vi "Clean up VI.vi"() -> ()   [LabVIEW 2013]
doc: "This .vi recenters the front panel \"pane\" to the origin, and adjusts the size of the window to fit the controls.\nIt also does the same with the block diagram."
uses:
  <vilib>/Utility/miscctls.llb/LVPointTypeDef.ctl
panel:
  in  "Cancel":bool
  # "Run this .vi and then click the frontpanel of\nthe .vi you wish to clean up."
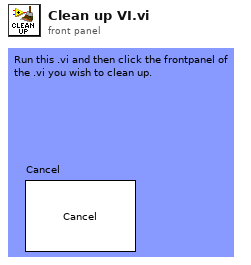
[diagram p1: front panel]
types:
  T1 = typedef "LVPointTypeDef.ctl" = cluster{"Horizontal":i16, "Vertical":i16}
  T2 = typedef "LVRectTypeDef.ctl" = cluster{"Left":i16, "Top":i16, "Right":i16, "Bottom":i16}
  T3 = enum32{"invalid VI type", "Standard VI", "Control VI", "Global VI", "Polymorphic VI", "Configuration VI", "SubSystem", "Facade VI", "Method VI", "Statechart Diagram VI"}
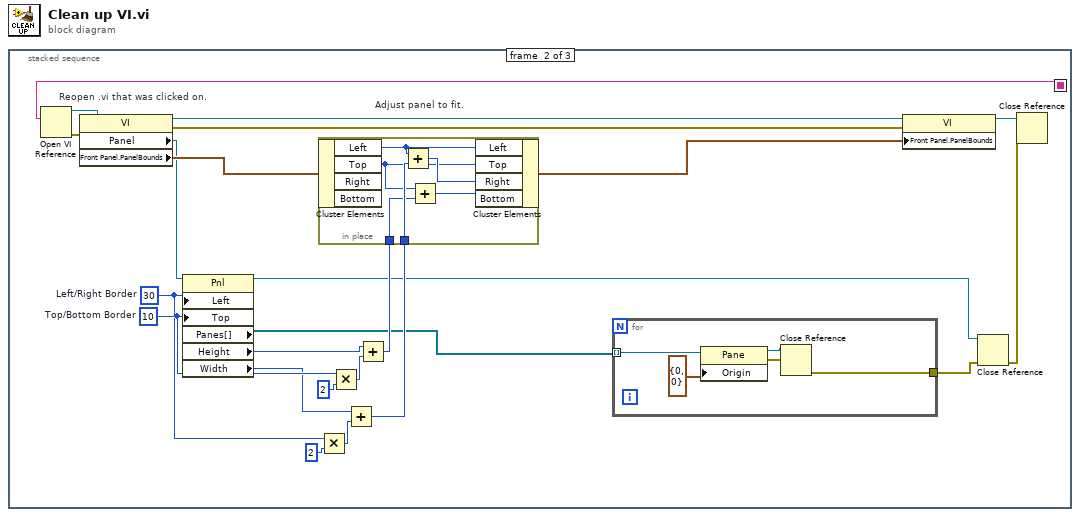
[diagram p0: block diagram]
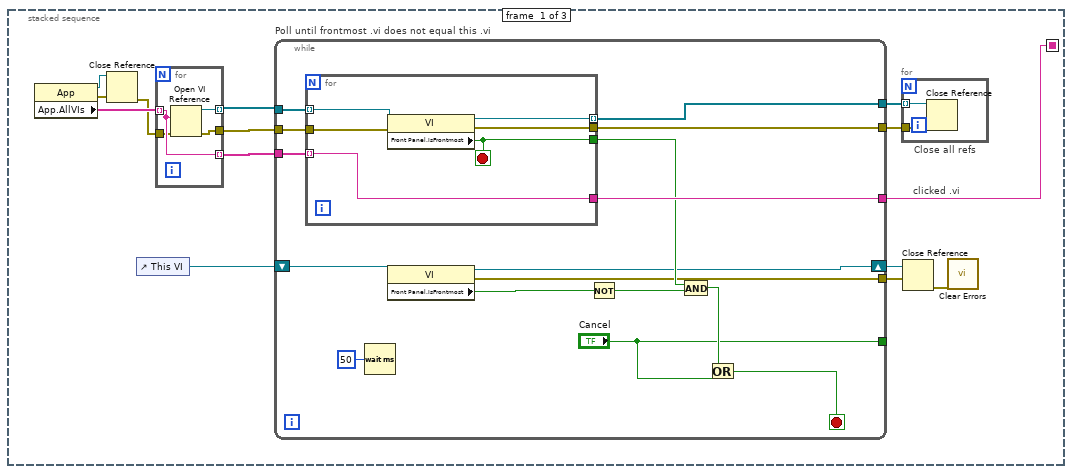
[diagram p2: hidden frame]
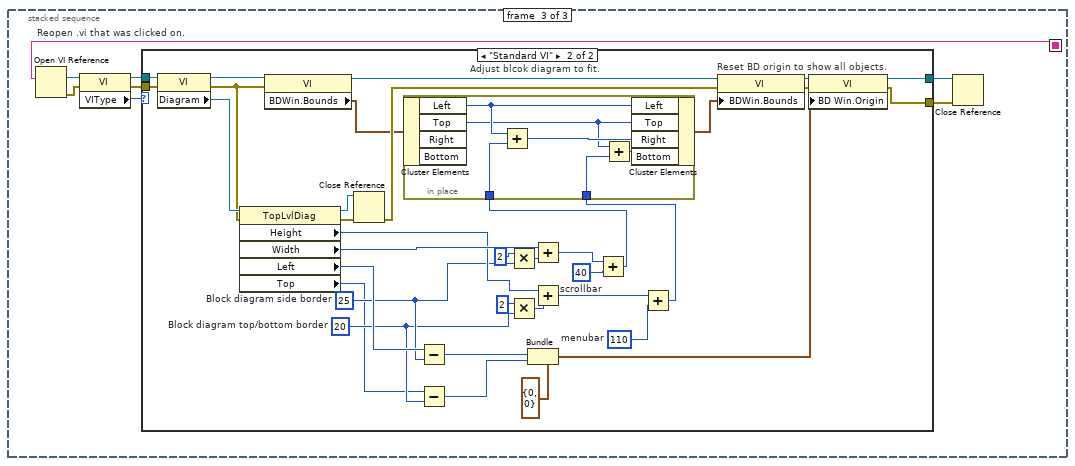
[diagram p3: hidden frame]
diagram:
  n1 = stacked-sequence {
    seq-local: [w13 _ _] -> [_ w43 w84]
    frame #0 {
      # "clicked .vi"
      n2 = property class="App"() -> (reference out=w5:refnum<vi>, error out=w6:errorcluster, "App.AllVIs"=w12:string[])  [unwired: 2 in]
      n3 = Close Reference(reference=w5, error in (no error)=w6) -> (error out=w4:errorcluster)
      n4 = control-ref of="This VI"() -> (w14:refnum<vi>)
      n5 = for {
        tunnel: w12 -> [w18] mode=indexing
        tunnel: [w20] -> w11 mode=indexing
        tunnel: [w19] -> w8
        tunnel: [w18] -> w7 mode=indexing
        tunnel: w4 -> [w17]
        n6 = Open VI Reference(vi path=w18, error in (no error)=w17) -> (vi reference=w20:refnum<vi>, error out=w19:errorcluster)  [unwired: 1 in, 3 out]
      }
      n7 = while "Poll until frontmost .vi does not equal this .vi" {
        tunnel: w11 -> [w36]
        tunnel: [w34] -> w13
        tunnel: ["Cancel"] -> _
        tunnel: [w26] -> w10
        tunnel: [w25] -> w9
        tunnel: w8 -> [w24]
        tunnel: w7 -> [w23]
        tunnel: [w22] -> w3
        shift-right: [w21] -> w2
        shift-left: w14 -> [w35]
        stop <- w32 stop-if-true
        n8 = for {
          tunnel: w36 -> [w41] mode=indexing
          tunnel: [w37] -> w34
          tunnel: [w42] -> w30
          tunnel: [w40] -> w26 mode=indexing
          tunnel: [w39] -> w25
          tunnel: w24 -> [w38]
          tunnel: w23 -> [w37] mode=indexing
          stop <- w42 stop-if-true
          n9 = property class="VI"(reference=w41, error in=w38) -> (reference out=w40:refnum<vi>, error out=w39:errorcluster, "Front Panel.IsFrontmost"=w42:bool)
        }
        n10 = Wait (ms)(milliseconds to wait=u32 50) -> ()  [unwired: 1 out]
        n11 = property class="VI"(reference=w35) -> (reference out=w21:refnum<vi>, error out=w22:errorcluster, "Front Panel.IsFrontmost"=w29:bool)  [unwired: 1 in]
        n12 = Not(x=w29) -> (.not. x?=w28:bool)
        n13 = And(x=w30, y=w28) -> (x .and. y?=w31:bool)
        n14 = Or(x=w31, y="Cancel") -> (x .or. y?=w32:bool)
      }
      n15 = for "Close all refs" {
        tunnel: w10 -> [w16] mode=indexing
        tunnel: w9 -> [w15]
        n16 = Close Reference(reference=w16, error in (no error)=w15) -> ()  [unwired: 1 out]
      }
      n17 = Close Reference(reference=w2, error in (no error)=w3) -> (error out=w1:errorcluster)
      n18 = call <vilib>:"Clear Errors.vi"("error in (no error)"=w1) -> ()  [unwired: 7 out]
    }
    frame #1 {
      w59 = 10  # Top/Bottom Border
      w54 = 30  # Left/Right Border
      # "Adjust panel to fit."
      # "Reopen .vi that was clicked on."
      n19 = Open VI Reference(vi path=w43) -> (vi reference=w44:refnum<vi>, error out=w45:errorcluster)  [unwired: 2 in, 3 out]
      n20 = property class="VI"(reference=w44, error in=w45) -> (reference out=w61:refnum<vi>, error out=w62:errorcluster, "Panel"=w46:refnum<vi>, "Front Panel.PanelBounds"=w50:T2)
      n21 = property class="Pnl"(reference=w46, "Left"=w54, "Top"=w59) -> (reference out=w49:refnum<vi>, "Panes[]"=w47:refnum<vi>[], "Height"=w58:u32, "Width"=w51:u32)  [unwired: 1 in, 1 out]
      n22 = Multiply(x=w54, y=2 ("Position:Left")) -> (x*y=w53:i32)
      n23 = Multiply(x=w59, y=2 ("Position:Left")) -> (x*y=w57:i32)
      n24 = Add(x=w51, y=w53) -> (x+y=w52:u32)
      n25 = Add(x=w58, y=w57) -> (x+y=w60:u32)
      n26 = in-place {
        in-place-border: w52 -> [w70]
        in-place-border: w60 -> [w69]
        n27 = in-place-cluster #1(w50) -> ("Left"=w67:i16, "Top"=w66:i16)  [unwired: 2 out]
        n28 = Add(x=w67, y=w70) -> (x+y=w71:u32)
        n29 = Add(x=w66, y=w69) -> (x+y=w68:u32)
        n30 = in-place-cluster #1("Left"=w67, "Top"=w66, "Right"=w71, "Bottom"=w68) -> (w63:T2)
      }
      n31 = for {
        tunnel: w47 -> [w76] mode=indexing
        tunnel: [w72] -> w48
        n32 = property class="Pane"(reference=w76, "Origin"=T1 {"Horizontal"=0, "Vertical"=0}) -> (reference out=w74:refnum<vi>, error out=w73:errorcluster)  [unwired: 1 in]
        n33 = Close Reference(reference=w74, error in (no error)=w73) -> (error out=w72:errorcluster)
      }
      n34 = property class="VI"(reference=w61, error in=w62, "Front Panel.PanelBounds"=w63) -> (reference out=w64:refnum<vi>)  [unwired: 1 out]
      n35 = Close Reference(reference=w49, error in (no error)=w48) -> (error out=w65:errorcluster)
      n36 = Close Reference(reference=w64, error in (no error)=w65) -> ()  [unwired: 1 out]
    }
    frame #2 {
      # "Reopen .vi that was clicked on."
      n37 = Open VI Reference(vi path=w84) -> (vi reference=w81:refnum<vi>, error out=w80:errorcluster)  [unwired: 2 in, 3 out]
      n38 = property class="VI"(reference=w81, error in=w80) -> (reference out=w78:refnum<vi>, error out=w79:errorcluster, "VIType"=w77:T3)
      n39 = case shown="\"Standard VI\"" w77 {
        tunnel: [w86 w99] -> w83
        tunnel: [w85 w98] -> w82
        tunnel: w79 -> [w86 w88]
        tunnel: w78 -> [w85 w87]
        frame Default {
          # "VI's with no diagrams."
        }
        frame "Standard VI" {
          w104 = u32 40  # scrollbar
          w106 = u32 110  # menubar
          w92 = i16 20  # Block diagram top/bottom border
          w96 = i16 25  # Block diagram side border
          # "Reset BD origin to show all objects."
          # "Adjust blcok diagram to fit."
          n40 = property class="VI"(reference=w87, error in=w88) -> (reference out=w118:refnum<vi>, error out=w117:errorcluster, "Diagram"=w121:refnum<vi>)
          n41 = property class="TopLvlDiag"(reference=w121, error in=w117) -> (reference out=w119:refnum<vi>, error out=w89:errorcluster, "Height"=w108:u32, "Width"=w113:u32, "Left"=w97:i32, "Top"=w91:i32)
          n42 = property class="VI"(reference=w118, error in=w117) -> (reference out=w116:refnum<vi>, "BDWin.Bounds"=w115:T2)  [unwired: 1 out]
          n43 = Close Reference(reference=w119, error in (no error)=w89) -> (error out=w120:errorcluster)
          n44 = Subtract(x=w97, y=w96) -> (x-y=w94:i32)
          n45 = Subtract(x=w91, y=w92) -> (x-y=w90:i32)
          n46 = Multiply(x=i16 2, y=w96) -> (x*y=w112:i16)
          n47 = Multiply(x=i16 2, y=w92) -> (x*y=w109:i16)
          n48 = Bundle(cluster=T1 {"Horizontal"=0, "Vertical"=0} ("Block Diagram Window:Origin"), "Horizontal"=w94, "Vertical"=w90) -> (w93:T1)
          n49 = Add(x=w113, y=w112) -> (x+y=w103:u32)
          n50 = Add(x=w108, y=w109) -> (x+y=w107:u32)
          n51 = Add(x=w103, y=w104) -> (x+y=w102:u32)
          n52 = Add(x=w107, y=w106) -> (x+y=w105:u32)
          n53 = in-place {
            in-place-border: w102 -> [w126]
            in-place-border: w105 -> [w122]
            n54 = in-place-cluster #2(w115) -> ("Left"=w124:i16, "Top"=w123:i16)  [unwired: 2 out]
            n55 = Add(x=w124, y=w126) -> (x+y=w127:u32)
            n56 = Add(x=w123, y=w122) -> (x+y=w125:u32)
            n57 = in-place-cluster #2("Left"=w124, "Top"=w123, "Right"=w127, "Bottom"=w125) -> (w114:T2)
          }
          n58 = property class="VI"(reference=w116, error in=w120, "BDWin.Bounds"=w114) -> (reference out=w101:refnum<vi>, error out=w100:errorcluster)
          n59 = property class="VI"(reference=w101, error in=w100, "BD Win.Origin"=w93) -> (reference out=w98:refnum<vi>, error out=w99:errorcluster)
        }
      }
      n60 = Close Reference(reference=w82, error in (no error)=w83) -> ()  [unwired: 1 out]
    }
  }
